vi "RS232ComPort WritePortInfo.vi"(8 "error in (no error)":errorcluster, 9 "Channel":i32, 10 "Status":i8, 11 "RS232ComPort in":refnum<class "RS232ComPort.lvclass">) -> (0 "error out":errorcluster, 3 "RS232ComPort out":refnum<class "RS232ComPort.lvclass">)   [LabVIEW 2018, in "RS232ComPort.lvclass"]
doc: "Channel status\n-1 | Laser\n0 | Not in used so far\n0..127 | # of device initialising with @"
uses:
  RS232ComPort.lvclass
  RS232ComPort.lvclass/RS232ComPort.ctl
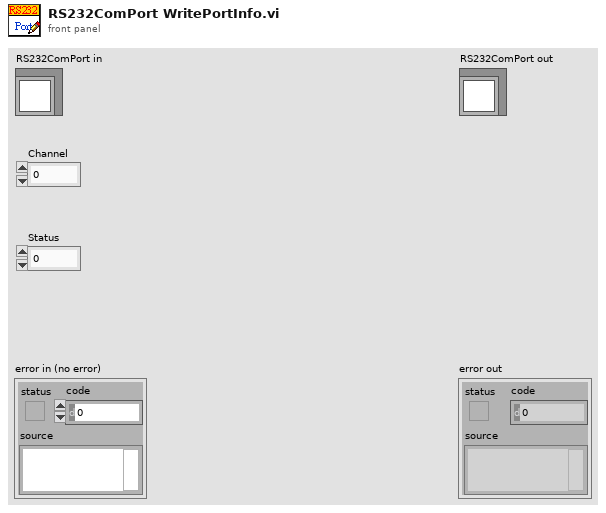
[diagram p1: front panel]
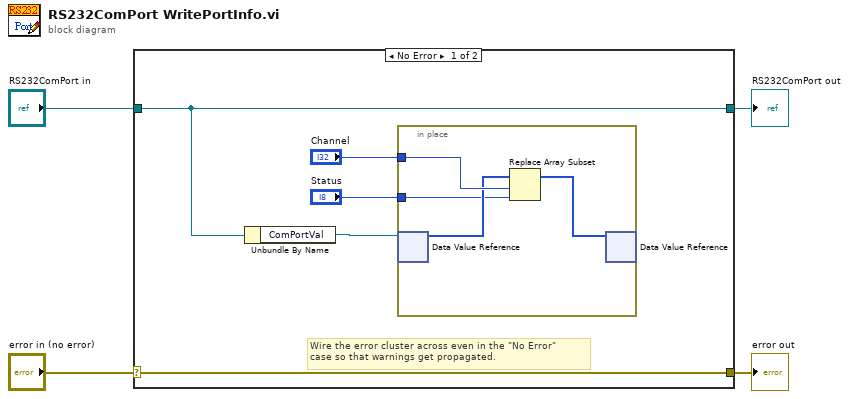
[diagram p0: block diagram]
diagram:
  n1 = case shown="No Error" "error in (no error)" {
    selector: "error in (no error)" -> [w9 w15]
    tunnel: [w9 w15] -> w3
    tunnel: [w8 w14] -> w1
    tunnel: "RS232ComPort in" -> [w8 w14]
    frame No Error {
      # "Wire the error cluster across even in the \"No Error\"\ncase so that warnings get propagated."
      n2 = Unbundle By Name(w8) -> ("ComPortVal"=w7:refnum<data-value>)
      n3 = in-place {
        in-place-border: "Channel" -> [w13]
        in-place-border: "Status" -> [w10]
        n4 = in-place-dvr #1(w7) -> (w11:i8[])  [unwired: 1 out]
        n5 = Replace Array Subset(array=w11, new element=w10, index=w13) -> (w12:i8[])
        n6 = in-place-dvr #1(w12) -> ()  [unwired: 2 out]
      }
    }
    frame Error {
    }
  }
  "error out" <- w3
  "RS232ComPort out" <- w1
